vi "RD_result.vi"(8 "lower limit":dbl=2.1 format="%#_13g", 9 "upper limit":dbl, 10 "name":string="123.txt", 11 "base path":path) -> (0 "左邊結果":bool, 1 "右邊結果":bool, 2 "左邊結果":string, 3 "右邊結果":string, 4 "R data":T1, 6 "L data":T1)   [LabVIEW 2019]
uses:
  <vilib>/regexp/Match Regular Expression.xnode
panel:
  out "左邊NG":bool[](array[boolean])
  out "右邊NG":bool[](array[boolean])
  out "前半段字數":i32
  out "Array 2":bool[](array[boolean])
  out "appended path":path
  out "text":string
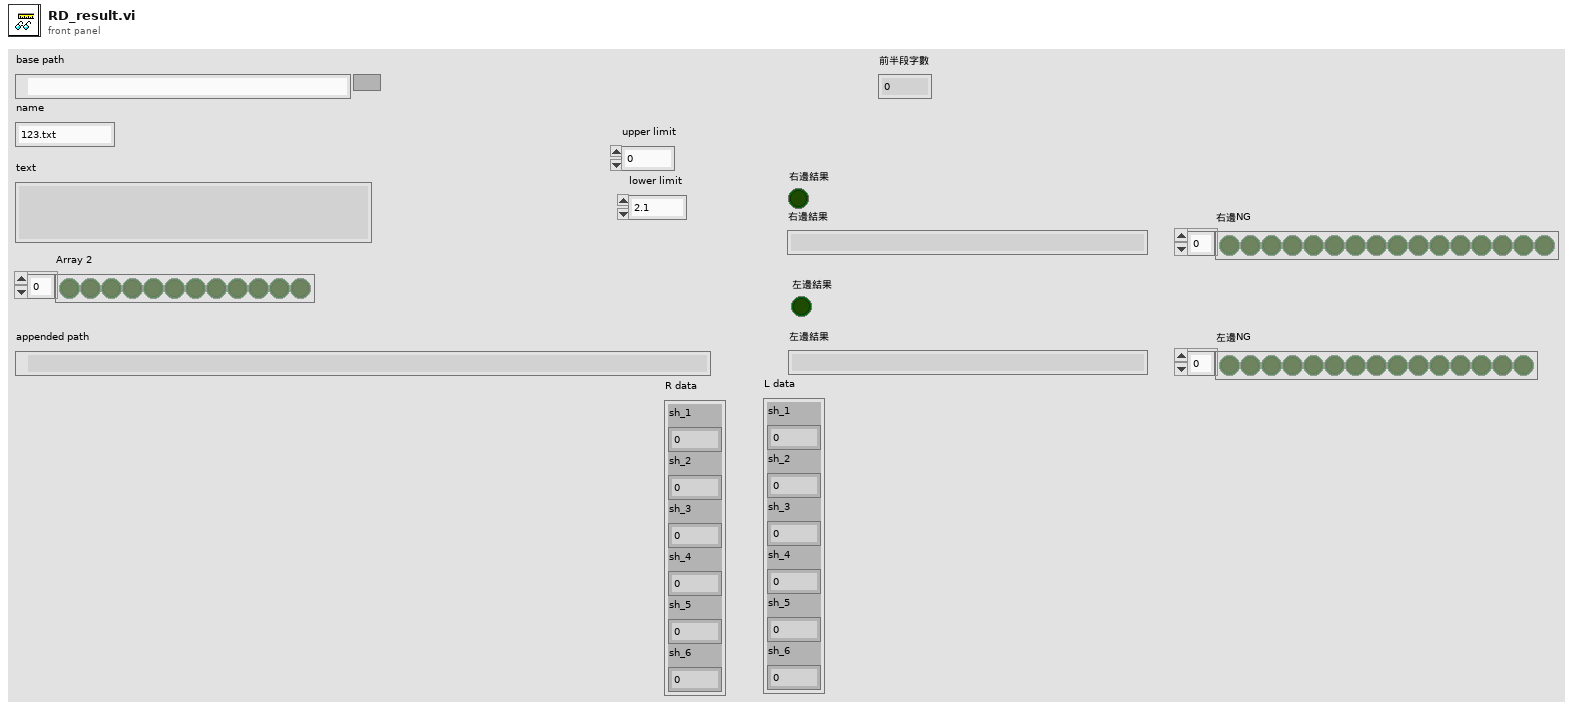
[diagram p1: front panel]
types:
  T1 = cluster{"sh_1":dbl, "sh_2":dbl, "sh_3":dbl, "sh_4":dbl, "sh_5":dbl, "sh_6":dbl}
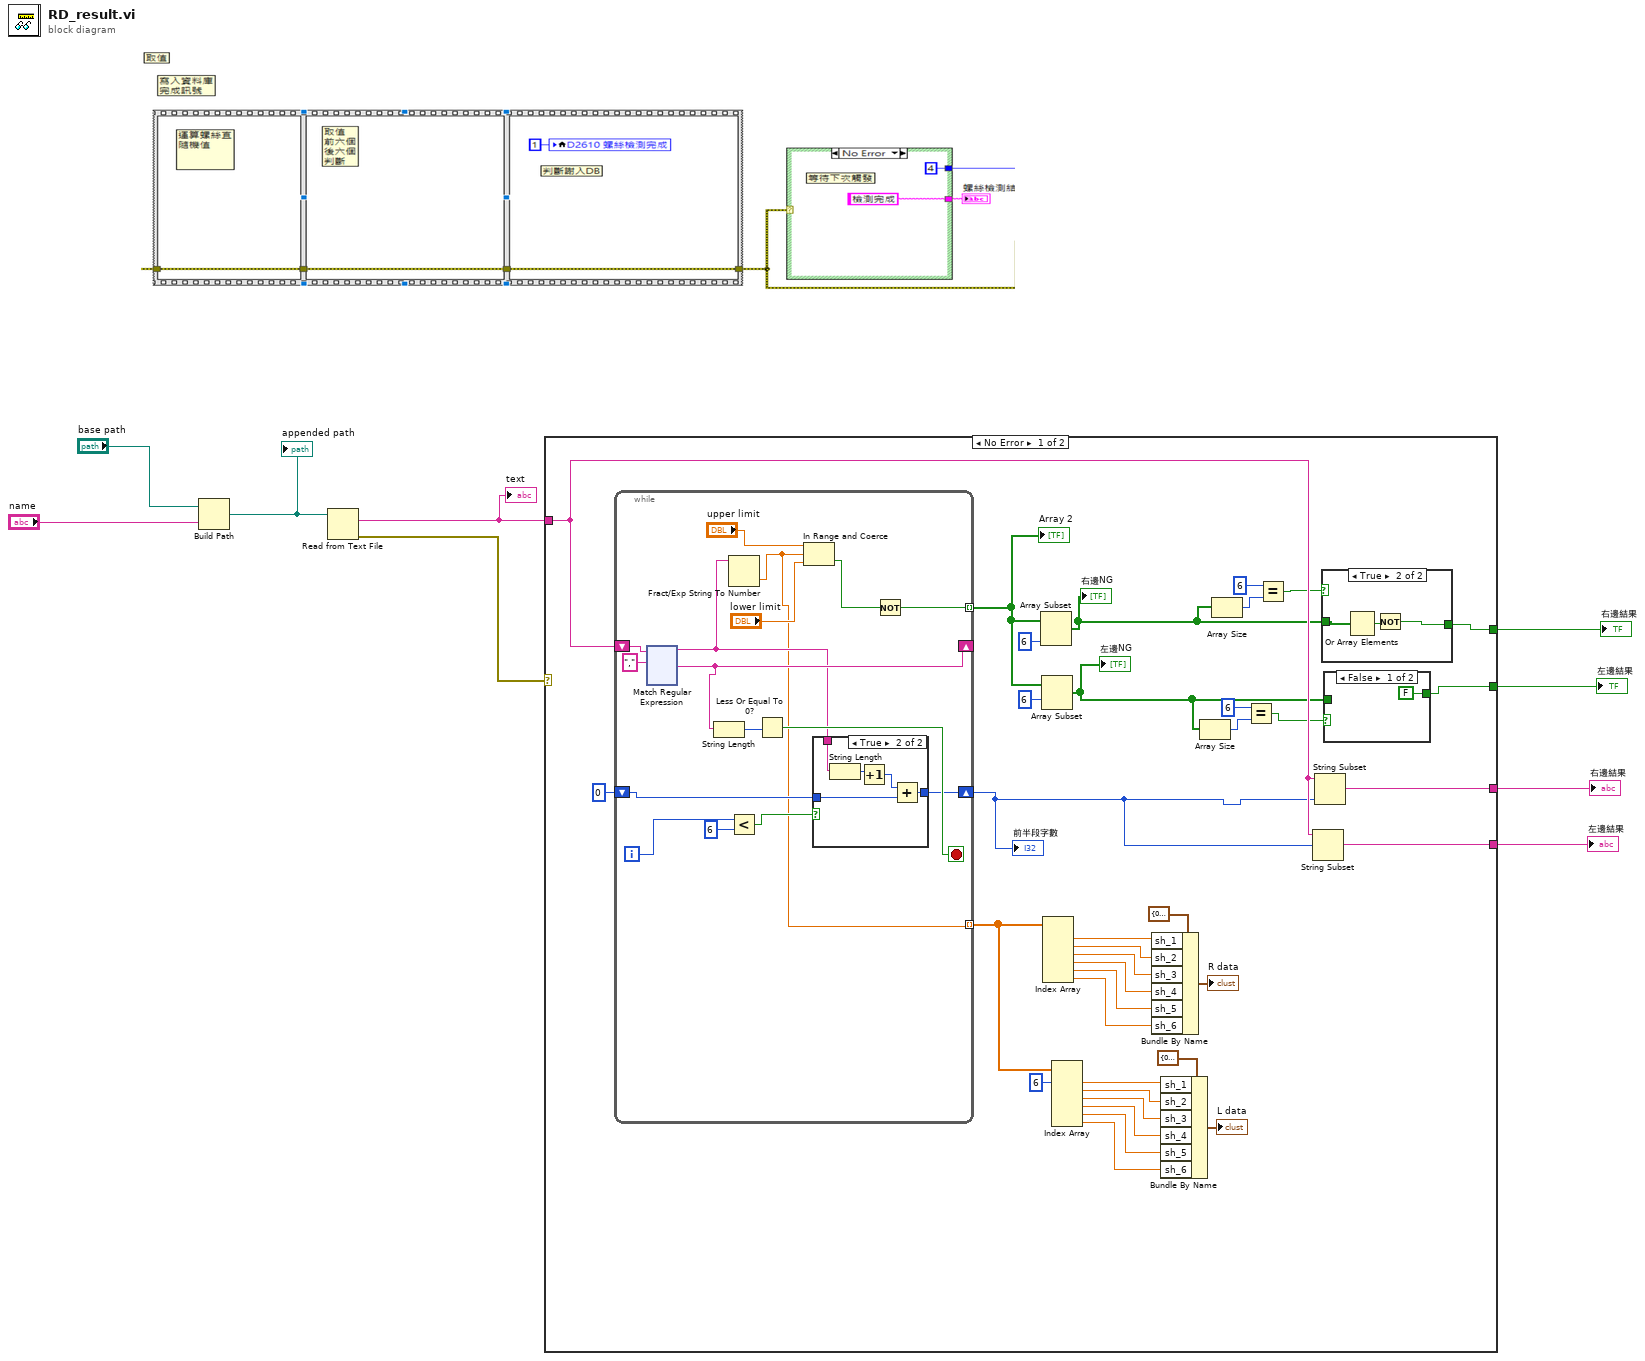
[diagram p0: block diagram]
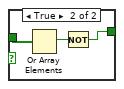
[diagram p2: hidden frame]
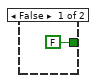
[diagram p3: hidden frame]
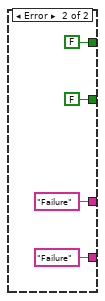
[diagram p5: hidden frame]
diagram:
  n1 = Build Path(base path="base path", name or relative path="name") -> (appended path=w9:path)
  "appended path" <- w9
  n2 = Read from Text File(file (use dialog)=w9) -> (text=w3:string, error out=w4:errorcluster)  [unwired: 3 in, 2 out]
  "text" <- w3
  n3 = case shown="No Error" w4 {
    tunnel: [w44 "Failure"] -> w8
    tunnel: w3 -> [w43 _]
    tunnel: [w42 "Failure"] -> w7
    tunnel: [w38 FALSE] -> w6
    tunnel: [w37 FALSE] -> w5
    frame No Error {
      n4 = while {
        shift-right: [w67] -> _
        shift-left: w43 -> [w68]
        tunnel: [w55] -> w40 mode=indexing
        shift-right: [w61] -> w28
        shift-left: 0 -> [w60]
        tunnel: [w54] -> w13 mode=indexing
        i -> [w64]
        stop <- w65 stop-if-true
        n5 = xnode "Match Regular Expression"("input string"=w68, "regular expression"=",") -> ("before match"=w59:string, "after match"=w67:string)  [unwired: 4 in, 3 out]
        n6 = String Length(string=w67) -> (length=w66:i32)
        n7 = Fract/Exp String To Number(string=w59) -> (number=w54:dbl)  [unwired: 3 in, 1 out]
        n8 = Less?(x=w64, y=6) -> (x < y?=w62:bool)
        n9 = Less Or Equal To 0?(x=w66) -> (x <= 0?=w65:bool)
        n10 = In Range and Coerce(upper limit="upper limit", x=w54, lower limit="lower limit") -> (In Range?=w56:bool)  [unwired: 1 out]
        n11 = case shown="True" w62 {
          tunnel: w59 -> [_ w75]
          tunnel: [w70 w72] -> w61
          tunnel: w60 -> [w70 w71]
          frame False {
          }
          frame True {
            n12 = String Length(string=w75) -> (length=w74:i32)
            n13 = Increment(x=w74) -> (x+1=w73:i32)
            n14 = Add(x=w73, y=w71) -> (x+y=w72:i32)
          }
        }
        n15 = Not(x=w56) -> (.not. x?=w55:bool)
      }
      "Array 2" <- w40
      "前半段字數" <- w28
      n16 = Array Subset(array=w40, length=6) -> (w35:bool[])  [unwired: 1 in]
      "右邊NG" <- w35
      n17 = Array Subset(array=w40, index=6 ("length")) -> (w30:bool[])  [unwired: 1 in]
      "左邊NG" <- w30
      n18 = Index Array(array=w13) -> (element #1=w22:dbl, element #2=w23:dbl, element #3=w24:dbl, element #4=w25:dbl, element #5=w26:dbl, element #6=w27:dbl)  [unwired: 6 in]
      n19 = Index Array(array=w13, index #1=6 ("index")) -> (element #1=w19:dbl, element #2=w18:dbl, element #3=w17:dbl, element #4=w16:dbl, element #5=w15:dbl, element #6=w14:dbl)  [unwired: 5 in]
      n20 = Bundle By Name(cluster=T1 {"sh_1"=0.0, "sh_2"=0.0, "sh_3"=0.0, "sh_4"=0.0, "sh_5"=0.0, "sh_6"=0.0}, "sh_1"=w22, "sh_2"=w23, "sh_3"=w24, "sh_4"=w25, "sh_5"=w26, "sh_6"=w27) -> (→"R data":T1)
      n21 = Bundle By Name(cluster=T1 {"sh_1"=0.0, "sh_2"=0.0, "sh_3"=0.0, "sh_4"=0.0, "sh_5"=0.0, "sh_6"=0.0}, "sh_1"=w19, "sh_2"=w18, "sh_3"=w17, "sh_4"=w16, "sh_5"=w15, "sh_6"=w14) -> (→"L data":T1)
      n22 = Array Size(array=w30) -> (size(s)=w32:i32)
      n23 = Array Size(array=w35) -> (size(s)=w34:i32)
      n24 = Equal?(x=6, y=w32) -> (x = y?=w29:bool)
      n25 = Equal?(x=6, y=w34) -> (x = y?=w36:bool)
      n26 = String Subset(string=w43, offset (0)=w28) -> (substring=w42:string)  [unwired: 1 in]
      n27 = String Subset(string=w43, length (rest)=w28) -> (substring=w44:string)  [unwired: 1 in]
      n28 = case shown="True" w36 {
        tunnel: w35 -> [_ w53]
        tunnel: [FALSE w51] -> w38
        frame False {
        }
        frame True {
          n29 = Or Array Elements(Boolean array=w53) -> (logical OR=w52:bool)
          n30 = Not(x=w52) -> (.not. x?=w51:bool)
        }
      }
      n31 = case shown="False" w29 {
        tunnel: [FALSE w49] -> w37
        tunnel: w30 -> [_ w47]
        frame False {
        }
        frame True {
          n32 = Or Array Elements(Boolean array=w47) -> (logical OR=w48:bool)
          n33 = Not(x=w48) -> (.not. x?=w49:bool)
        }
      }
    }
    frame Error {
    }
  }
  "右邊結果" <- w8
  "左邊結果" <- w7
  "右邊結果" <- w6
  "左邊結果" <- w5
